vi "AquisiçãoSinais.vi"(8 "error in":errorcluster, 11 "Analog":cluster{"Function":i32, "Channel":refnum<k21>}[](array[cluster])) -> (0 "error out":errorcluster)   [LabVIEW 2019]
uses:
  <vilib>/DAQmx/read.llb/DAQmx Read (Analog 1D DBL 1Chan NSamp).vi
  <vilib>/Analysis/baseanly.llb/Mean (DBL).vi
  <vilib>/DAQmx/miscellaneous.llb/DAQmx Fill In Error Info.vi
  VariaveisTaskMedicao.vi
  <vilib>/Analysis/NI_AALBase.lvlib
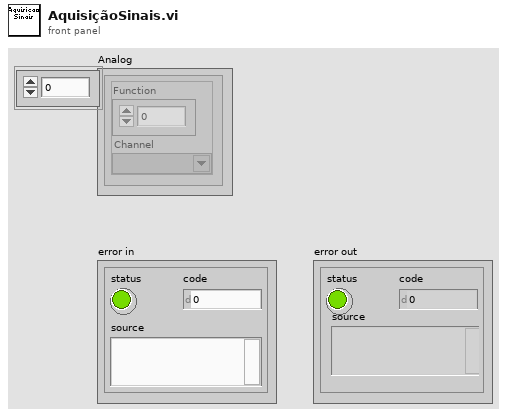
[diagram p1: front panel]
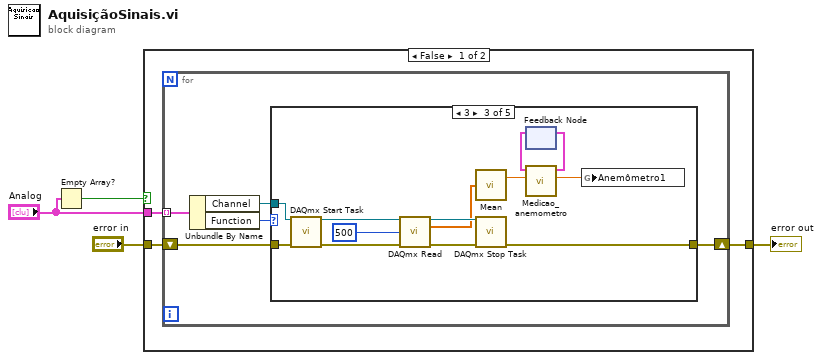
[diagram p0: block diagram]
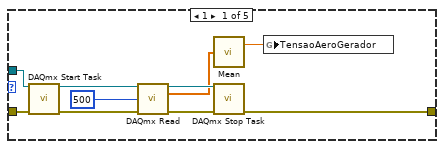
[diagram p2: hidden frame]
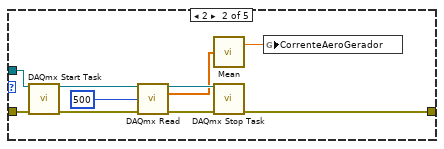
[diagram p3: hidden frame]
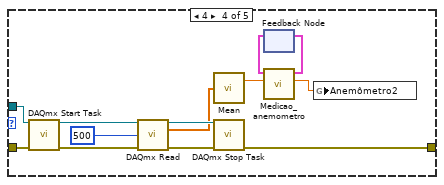
[diagram p4: hidden frame]
diagram:
  n1 = Empty Array?(array="Analog") -> (empty?=w2:bool)
  n2 = case shown="False" w2 {
    tunnel: "Analog" -> [w6 _]
    tunnel: [w5 w60] -> w1
    tunnel: "error in" -> [w7 w60]
    frame False {
      n3 = for {
        tunnel: w6 -> [w12] mode=indexing
        shift-right: [w10] -> w5
        shift-left: w7 -> [w9]
        n4 = Unbundle By Name(w12) -> ("Channel"=w8:refnum<k21>, "Function"=w11:i32)
        n5 = case shown="3" w11 {
          tunnel: w9 -> [w20 w30 w43 w56 w59]
          tunnel: w8 -> [w22 w32 w45 w58 _]
          tunnel: [w16 w26 w39 w52 w59] -> w10
          frame 1 {
            n6 = call <vilib>:"DAQmx Start Task.vi"("task/channels in"=w22, "error in"=w20) -> ("task out"=w21:refnum<k21>, "error out"=w19:errorcluster)  [unwired: 12 in]
            n7 = call-poly <vilib>:"DAQmx Read.vi"("task/channels in"=w21, "number of samples per channel"=500, "error in"=w19) -> ("task out"=w18:refnum<k21>, "data"=w15:dbl[], "error out"=w17:errorcluster)  [unwired: 10 in]
            n8 = call-poly <vilib>:"Mean.vi"("X"=w15) -> ("mean"=w13:dbl)  [unwired: 1 out]
            n9 = call <vilib>:"DAQmx Stop Task.vi"("task/channels in"=w18, "error in"=w17) -> ("error out"=w16:errorcluster)  [unwired: 12 in, 1 out]
            n10 = global write "VariaveisTaskMedicao.vi" "TensaoAeroGerador"(w13) -> ()
          }
          frame 2 {
            n11 = call <vilib>:"DAQmx Start Task.vi"("task/channels in"=w32, "error in"=w30) -> ("task out"=w31:refnum<k21>, "error out"=w29:errorcluster)  [unwired: 12 in]
            n12 = call-poly <vilib>:"DAQmx Read.vi"("task/channels in"=w31, "number of samples per channel"=500, "error in"=w29) -> ("task out"=w28:refnum<k21>, "data"=w25:dbl[], "error out"=w27:errorcluster)  [unwired: 10 in]
            n13 = call-poly <vilib>:"Mean.vi"("X"=w25) -> ("mean"=w23:dbl)  [unwired: 1 out]
            n14 = call <vilib>:"DAQmx Stop Task.vi"("task/channels in"=w28, "error in"=w27) -> ("error out"=w26:errorcluster)  [unwired: 12 in, 1 out]
            n15 = global write "VariaveisTaskMedicao.vi" "CorrenteAeroGerador"(w23) -> ()
          }
          frame 3 {
            n16 = call <vilib>:"DAQmx Start Task.vi"("task/channels in"=w45, "error in"=w43) -> ("task out"=w44:refnum<k21>, "error out"=w42:errorcluster)  [unwired: 12 in]
            n17 = call-poly <vilib>:"DAQmx Read.vi"("task/channels in"=w44, "number of samples per channel"=500, "error in"=w42) -> ("task out"=w41:refnum<k21>, "data"=w38:dbl[], "error out"=w40:errorcluster)  [unwired: 10 in]
            n18 = call-poly <vilib>:"Mean.vi"("X"=w38) -> ("mean"=w34:dbl)  [unwired: 1 out]
            n19 = call <vilib>:"DAQmx Stop Task.vi"("task/channels in"=w41, "error in"=w40) -> ("error out"=w39:errorcluster)  [unwired: 12 in, 1 out]
            n20 = feedback #1() -> (w36:cluster{"GraphSenoide":i32[], "NivelAlto":bool})  [unwired: 1 in]
            n21 = call "Medicao_anemometro.vi"("Anemometro"=w34, "DadosGraphInp"=w36) -> ("Sinal"=w33:dbl, "DadosGraph"=w35:cluster{"GraphSenoide":i32[], "NivelAlto":bool})  [unwired: 8 in]
            n22 = feedback-in #1(w35) -> ()
            n23 = global write "VariaveisTaskMedicao.vi" "Anemômetro1"(w33) -> ()
          }
          frame 4 {
            n24 = call <vilib>:"DAQmx Start Task.vi"("task/channels in"=w58, "error in"=w56) -> ("task out"=w57:refnum<k21>, "error out"=w55:errorcluster)  [unwired: 12 in]
            n25 = call-poly <vilib>:"DAQmx Read.vi"("task/channels in"=w57, "number of samples per channel"=500, "error in"=w55) -> ("task out"=w54:refnum<k21>, "data"=w51:dbl[], "error out"=w53:errorcluster)  [unwired: 10 in]
            n26 = call-poly <vilib>:"Mean.vi"("X"=w51) -> ("mean"=w49:dbl)  [unwired: 1 out]
            n27 = call <vilib>:"DAQmx Stop Task.vi"("task/channels in"=w54, "error in"=w53) -> ("error out"=w52:errorcluster)  [unwired: 12 in, 1 out]
            n28 = feedback #2() -> (w47:cluster{"GraphSenoide":i32[], "NivelAlto":bool})  [unwired: 1 in]
            n29 = call "Medicao_anemometro.vi"("Anemometro"=w49, "DadosGraphInp"=w47) -> ("Sinal"=w46:dbl, "DadosGraph"=w48:cluster{"GraphSenoide":i32[], "NivelAlto":bool})  [unwired: 8 in]
            n30 = feedback-in #2(w48) -> ()
            n31 = global write "VariaveisTaskMedicao.vi" "Anemômetro2"(w46) -> ()
          }
          frame Default {
          }
        }
      }
    }
    frame True {
    }
  }
  "error out" <- w1
